vi "load_collection.vi"(8 "error in (no error)":errorcluster, 10 "index":i32, 11 "AnalysisRAPS in":refnum<class "AnalysisRAPS.lvclass">) -> (0 "error out":errorcluster, 3 "AnalysisRAPS out":refnum<class "AnalysisRAPS.lvclass">)   [LabVIEW 2010, in "AnalysisRAPS.lvclass"]
uses:
  AnalysisRAPS.lvclass
  AnalysisRAPS.lvclass/AnalysisRAPS.ctl
  common/classes/Image/Image/Image.lvclass
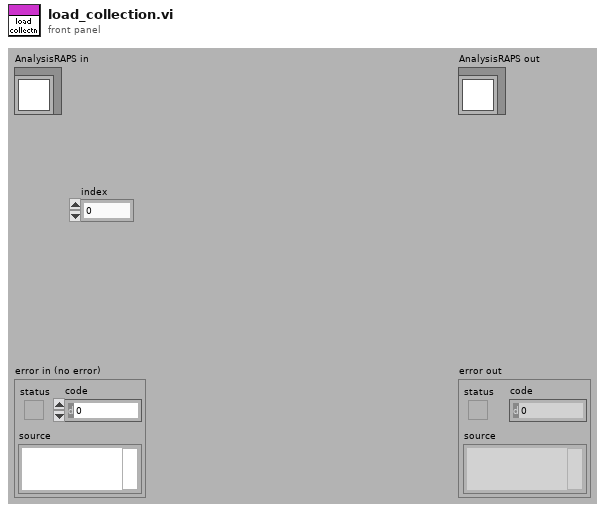
[diagram p1: front panel]
types:
  T1 = typedef "Image Type" = u32
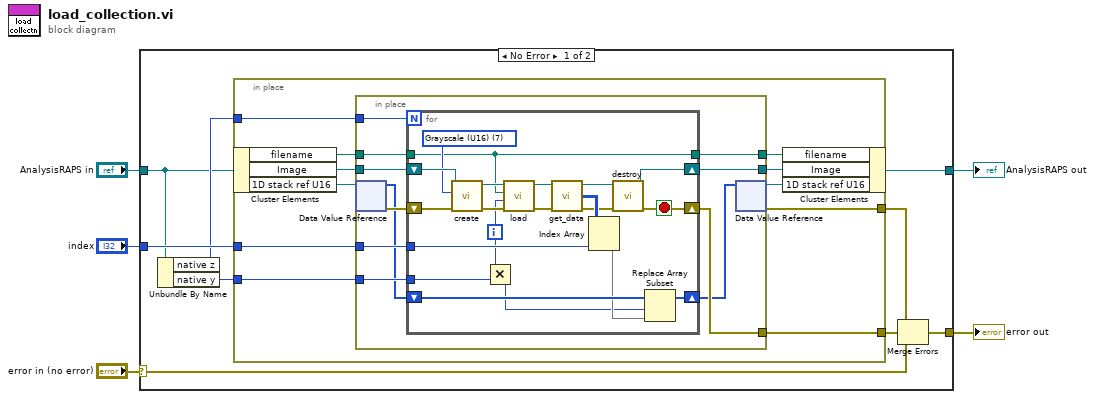
[diagram p0: block diagram]
diagram:
  n1 = case shown="No Error" "error in (no error)" {
    selector: "error in (no error)" -> [w6 w58]
    tunnel: [w12 w58] -> w4
    tunnel: [w7 w57] -> w2
    tunnel: "AnalysisRAPS in" -> [w8 w57]
    tunnel: "index" -> [w11 _]
    frame No Error {
      n2 = Unbundle By Name(w8) -> ("native z"=w10:i32, "native y"=w9:i32)
      n3 = in-place {
        in-place-border: [w25] -> w14
        in-place-border: [w24] -> w13
        in-place-border: w11 -> [w23]
        in-place-border: w10 -> [w22]
        in-place-border: w9 -> [w21]
        n4 = in-place-cluster #1(w8) -> ("filename"=w16:path, "Image"=w20:refnum<class "Image.lvclass">, "1D stack ref U16"=w18:refnum<data-value>)
        n5 = in-place {
          in-place-border: [w35] -> w24
          in-place-border: w20 -> [w36]
          in-place-border: w22 -> [w32]
          in-place-border: w23 -> [w33]
          in-place-border: w21 -> [w31]
          in-place-border: [w30] -> w19
          in-place-border: w16 -> [w28]
          in-place-border: [w27] -> w15
          n6 = in-place-dvr #2(w18) -> (w26:u16[], w34:errorcluster)
          n7 = for {
            N: w32 -> [_]
            shift-right: [w39] -> w35
            shift-left: w34 -> [w48]
            shift-right: [w37] -> w30
            shift-left: w36 -> [w49]
            tunnel: w33 -> [w55]
            shift-right: [w53] -> w29
            shift-left: w26 -> [w54]
            tunnel: w31 -> [w51]
            tunnel: w28 -> [w43]
            tunnel: [w43] -> w27
            i -> [w44]
            stop <- w39 stop-if-true
            w47 = T1 7 items=["Grayscale (U8)", "Grayscale (I16)", "Grayscale (SGL)", "Complex (CSG)", "RGB (U32)", "HSL (U32)", "RGB (U64)", "Grayscale (U16)"] ("Image Type")
            n8 = call "create.vi"("error in (no error)"=w48, "Image Type"=w47, "Image in"=w49) -> ("error out"=w46:errorcluster, "Image out"=w45:refnum<class "Image.lvclass">)  [unwired: 7 in]
            n9 = Multiply(x=w44, y=w51) -> (x*y=w50:i32)
            n10 = call-dynamic "load.vi"("error in (no error)"=w46, "page"=w44, "Path"=w43, "Image in"=w45) -> ("error out"=w41:errorcluster, "Image out"=w42:refnum<class "Image.lvclass">)  [unwired: 4 in, 2 out]
            n11 = call-dynamic "get_data.vi"("Image in"=w42, "error in (no error)"=w41) -> ("Image out"=w38:refnum<class "Image.lvclass">, "Image Pixels (U16)"=w56:u16[][], "error out"=w40:errorcluster)  [unwired: 5 in, 6 out]
            n12 = Index Array(array=w56, index (col)=w55) -> (element=w52:u16[])  [unwired: 1 in]
            n13 = call-dynamic "destroy.vi"("error in (no error)"=w40, "Image in"=w38) -> ("error out"=w39:errorcluster, "Image out"=w37:refnum<class "Image.lvclass">)  [unwired: 8 in]
            n14 = Replace Array Subset(array=w54, new element=w52, index=w50) -> (w53:u16[])
          }
          n15 = in-place-dvr #2(w29) -> (w17:refnum<data-value>, w25:errorcluster)
        }
        n16 = in-place-cluster #1("filename"=w15, "Image"=w19, "1D stack ref U16"=w17) -> (w7:refnum<class "AnalysisRAPS.lvclass">)
      }
      n17 = Merge Errors(w14, w13, w6) -> (w12:errorcluster)
    }
    frame Error {
    }
  }
  "error out" <- w4
  "AnalysisRAPS out" <- w2
